vi "Set_DI.vi"(0 "reference in":refnum<class "Sig_DI_Simple.lvclass">, 5 "DI":bool, 11 "error in (no error)":errorcluster) -> (4 "reference out":refnum<class "Sig_DI_Simple.lvclass">, 15 "error out":errorcluster)   [LabVIEW 2019, in "Sig_DI_Simple.lvclass"]
uses:
  Sig_DI_Simple.lvclass
  D:/GIT H4000/H4000/src/Proccess_class/Proccess.lvclass
  Sig_DI_Simple.lvclass/Sig_DI_Simple.ctl
  Proccess_class/Proccess.lvclass/Proccess.ctl
  Proccess_class/Read TagName.vi
  Proccess_class/Read Logger.vi
  Logger_class/WriteEvent.vi
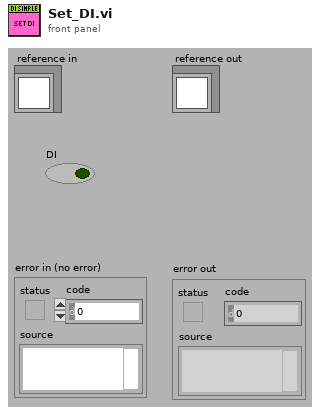
[diagram p1: front panel]
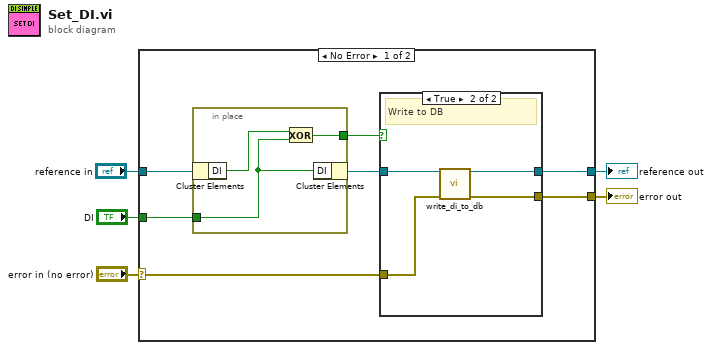
[diagram p0: block diagram]
diagram:
  n1 = case shown="No Error" "error in (no error)" {
    selector: "error in (no error)" -> [w12 w23]
    tunnel: [w9 w23] -> w4
    tunnel: [w10 w22] -> w2
    tunnel: "reference in" -> [w11 w22]
    tunnel: "DI" -> [w7 _]
    frame No Error {
      n2 = in-place {
        in-place-border: w7 -> [w21]
        in-place-border: [w20] -> w8
        n3 = in-place-cluster #1(w11) -> ("DI"=w19:bool)
        n4 = Exclusive Or(1:w21, 2:w19) -> (0:w20:bool)
        n5 = in-place-cluster #1("DI"=w21) -> (w6:refnum<class "Sig_DI_Simple.lvclass">)
      }
      n6 = case shown="True" w8 {
        tunnel: w6 -> [w14 w16]
        tunnel: [w14 w18] -> w10
        tunnel: w12 -> [w13 w15]
        tunnel: [w13 w17] -> w9
        frame False {
        }
        frame True {
          # "Write to DB"
          n7 = call "write_di_to_db.vi"("reference in"=w16, "error in (no error)"=w15) -> ("reference out"=w18:refnum<class "Sig_DI_Simple.lvclass">, "error out"=w17:errorcluster)  [unwired: 12 in]
        }
      }
    }
    frame Error {
    }
  }
  "error out" <- w4
  "reference out" <- w2
